vi "Simple TCP -사인파,삼각파 Server.vi"() -> ()   [LabVIEW 2018]
doc: "Demonstrates how to set up a basic TCP connection, send data to the specified port once a connection has been established, and terminate the connection once the data has been sent. This VI is designed to stop if the TCP connection is terminated. The data sent in this example is an array of random numbers."
panel:
  out "웨이브폼 그래프":dynamicdata(graph)
  in  "Client Closed":string="The client VI closed the connection."
  in  "Stop":bool
  # "Overview: Demonstrates the use of the TCP functions to initialize a TCP server that can send data to a client VI.\nInstructions:\n1. Run the VI.\n2. Open Simple TCP - Client.vi and follow the instructions on its front panel. Note that if you wait longer than 30 seconds to do this after running this VI, it will time out.\n3. Click Stop to stop the VI. Note that if you stop the client VI, this VI will stop automatically."
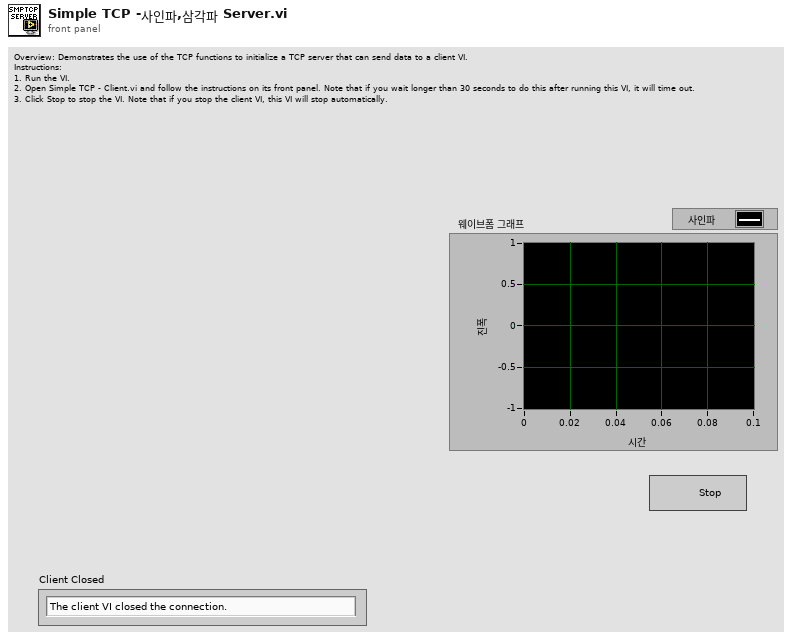
[diagram p1: front panel]
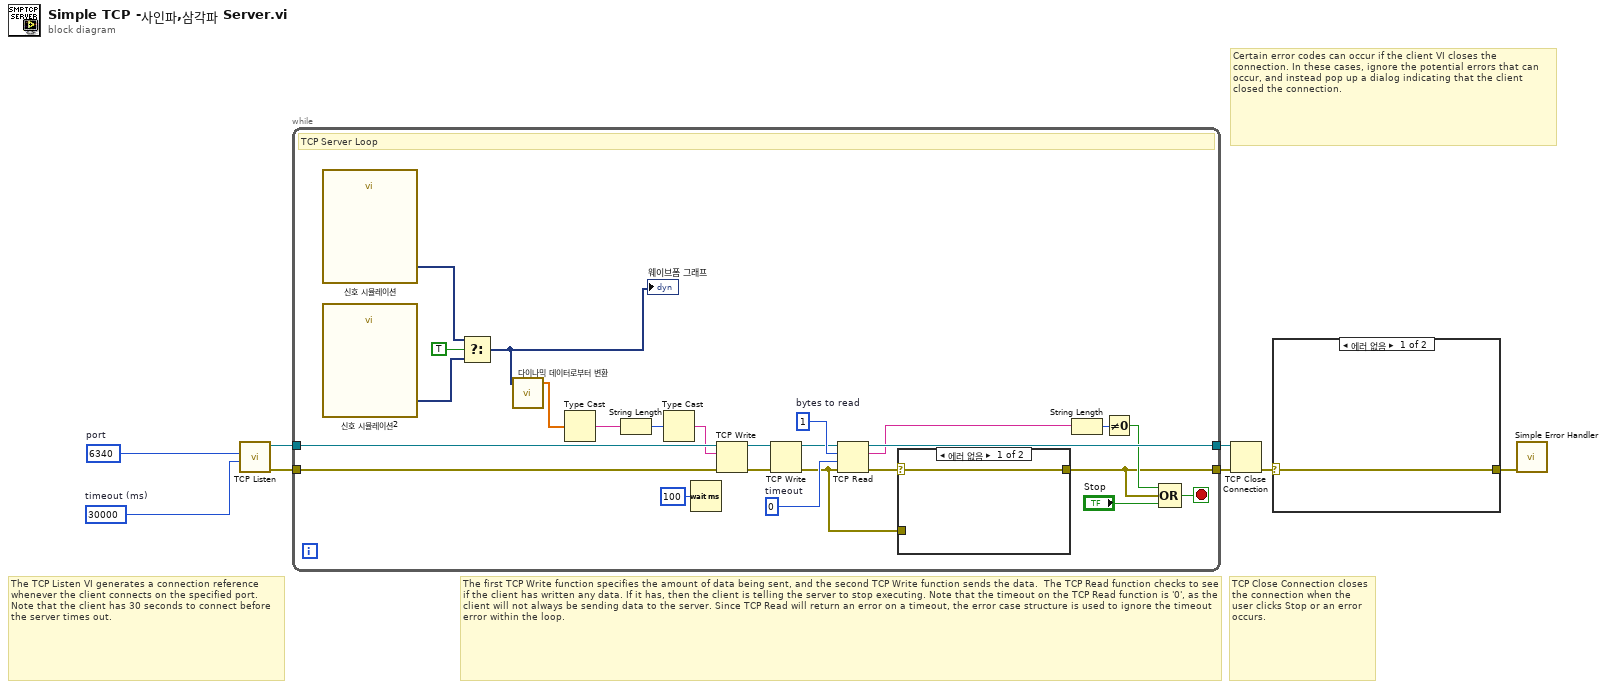
[diagram p0: block diagram]
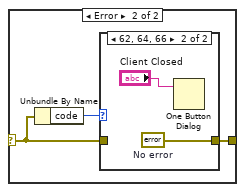
[diagram p2: hidden frame]
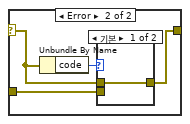
[diagram p4: hidden frame]
diagram:
  w1 = u16 6340  # port
  w2 = 30000  # timeout (ms)
  # "TCP Close Connection closes the connection when the user clicks Stop or an error occurs."
  # "The TCP Listen VI generates a connection reference whenever the client connects on the specified port. Note that the client has 30 seconds to connect before the server times out."
  # "Certain error codes can occur if the client VI closes the connection. In these cases, ignore the potential errors that can occur, and instead pop up a dialog indicating that the client closed the connection."
  # "The first TCP Write function specifies the amount of data being sent, and the second TCP Write function sends the data.  The TCP Read function checks to see if the client has written any data. If it has, then the client is telling the server to stop executing. Note that the timeout on the TCP Read function is '0', as the client will not always be sending data to the server. Since TCP Read will return an error on a timeout, the error case structure is used to ignore the timeout error within the loop."
  n1 = call <vilib>:"TCP Listen.vi"("timeout ms (wait forever: -1)"=w2, "port"=w1) -> ("error out"=w3:errorcluster, "connection ID"=w4:refnum<k5>)  [unwired: 5 in, 3 out]
  n2 = while {
    tunnel: [w16] -> w7
    tunnel: [w22] -> w8
    tunnel: w4 -> [w33]
    tunnel: w3 -> [w26]
    stop <- w27 stop-if-true
    w21 = 0  # timeout
    w24 = 1  # bytes to read
    # "TCP Server Loop"
    n3 = call "신호 시뮬레이션"() -> ("사인파"=w14:dynamicdata)  [unwired: 14 in, 1 out]
    n4 = call "신호 시뮬레이션2"() -> ("삼각파"=w13:dynamicdata)  [unwired: 14 in, 1 out]
    n5 = Select(t=w14, s=TRUE, f=w13) -> (s? t:f=w11:dynamicdata)
    "웨이브폼 그래프" <- w11
    n6 = call "다이나믹 데이터로부터 변환"("Dynamic Data Type"=w11) -> ("Array"=w10:dbl[])  [unwired: 3 in]
    n7 = Type Cast(x=w10) -> (*(type *) &x=w9:string)  [unwired: 1 out]
    n8 = String Length(string=w9) -> (length=w30:i32)
    n9 = Type Cast(x=w30) -> (*(type *) &x=w29:string)  [unwired: 1 out]
    n10 = Wait (ms)(milliseconds to wait=u32 100) -> ()  [unwired: 1 out]
    n11 = TCP Write(connection ID=w33, data in=w29, error in (no error)=w26) -> (connection ID out=w32:refnum<k5>, error out=w31:errorcluster)  [unwired: 2 out]
    n12 = TCP Write(connection ID=w32, error in (no error)=w31) -> (connection ID out=w23:refnum<k5>, error out=w15:errorcluster)  [unwired: 1 in, 2 out]
    n13 = TCP Read(connection ID=w23, bytes to read=w24, error in (no error)=w15, 9:w21) -> (connection ID out=w22:refnum<k5>, data out=w19:string, error out=w17:errorcluster)  [unwired: 1 out]
    n14 = case shown="에러 없음" w17 {
      selector: w17 -> [w34 w37]
      tunnel: [w34 w35] -> w16
      tunnel: w15 -> [_ w36]
      frame No Error {
      }
      frame Error {
        n15 = Unbundle By Name(w37) -> ("code"=w38:i32)
        n16 = case shown="기본" w38 {
          tunnel: w37 -> [w39 _]
          tunnel: w36 -> [_ w40]
          tunnel: [w39 w40] -> w35
          frame Default {
          }
          frame 56 {
          }
        }
      }
    }
    n17 = String Length(string=w19) -> (length=w20:i32)
    n18 = Not Equal To 0?(x=w20) -> (x != 0?=w18:bool)
    n19 = Compound Arithmetic op=OR(w18, w16, "Stop") -> (w27:bool)
  }
  n20 = TCP Close Connection(connection ID=w8, error in (no error)=w7) -> (error out=w6:errorcluster)  [unwired: 2 out]
  n21 = case shown="에러 없음" w6 {
    selector: w6 -> [w41 w43]
    tunnel: [w41 w42] -> w5
    frame No Error {
    }
    frame Error {
      n22 = Unbundle By Name(w43) -> ("code"=w44:i32)
      n23 = case shown="62, 64, 66" w44 {
        tunnel: w43 -> [w45 _]
        tunnel: [w45 w47] -> w42
        frame Default {
        }
        frame 62, 64, 66 {
          w47 = errorcluster {"status"=FALSE, "code"=0, "source"=""}  # No error
          n24 = One Button Dialog(message="Client Closed") -> ()  [unwired: 1 in, 1 out]
        }
      }
    }
  }
  n25 = call <vilib>:"Simple Error Handler.vi"("error in (no error)"=w5) -> ()  [unwired: 1 in, 8 out]
